vi "Music Visualizer Example.vi"() -> ()   [LabVIEW 2020]
uses:
  <vilib>/Analysis/5stat.llb/RMS (DBL).vi
  <vilib>/sound2/lvsound2.llb/Sound File Info (path).vi
  <vilib>/sound2/lvsound2.llb/Sound File Read Open.vi
  <vilib>/sound2/lvsound2.llb/Sound File Read (DBL).vi
  <vilib>/sound2/lvsound2.llb/Sound Output Write (DBL).vi
  <vilib>/Analysis/NI_AALPro.lvlib
  <vilib>/ptbypt/NI_PtbyPt.lvlib
panel:
  in  "Color Box":u32(colorbox)=5883391
  out "XY Graph":cluster{dbl[], dbl[]}[](graph)
  in  "Stop":bool
  in  "Buffer Size (samples)":i32=2048
  in  "Music File":path
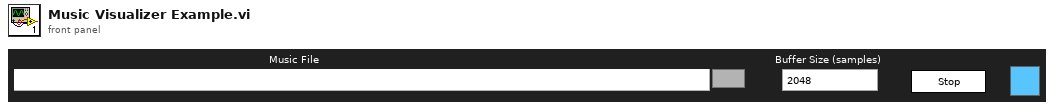
[diagram p1: front panel]
types:
  T1 = typedef "Sound Data Format.ctl" = cluster{"sample rate (S/s)":dbl, "number of channels":i32, "bits per sample":i32}
  T2 = typedef "Sound Output Task ID.ctl" = u32
  T3 = typedef "Sound File Refnum.ctl" = refnum<file>
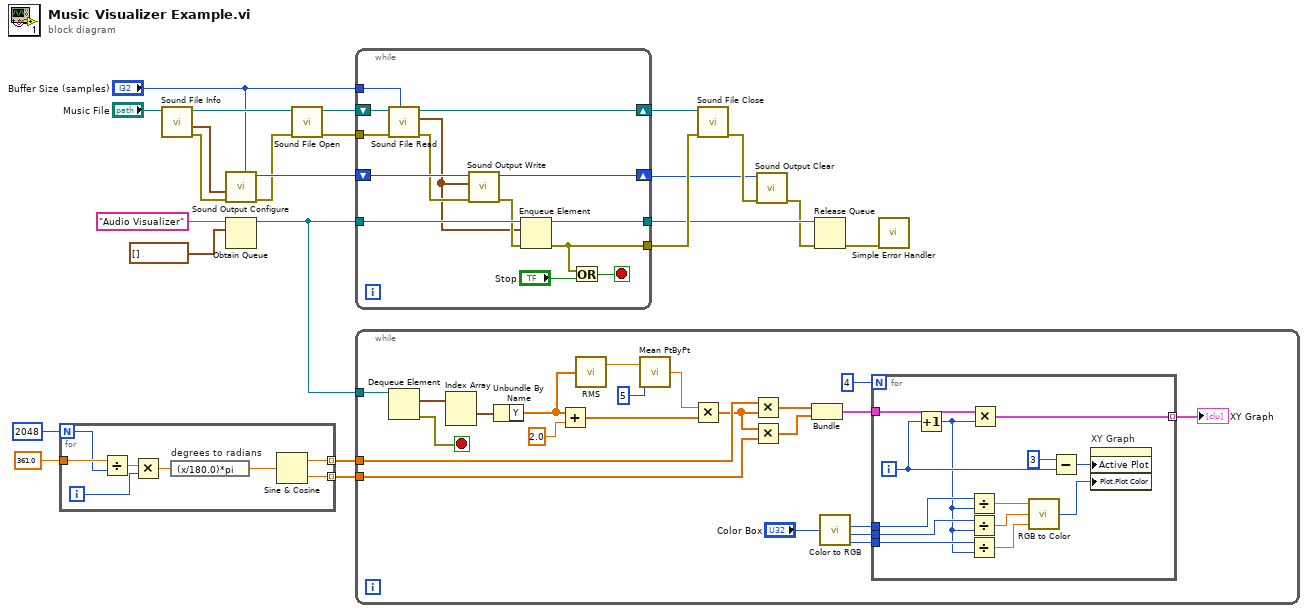
[diagram p0: block diagram]
diagram:
  n1 = for {
    N: 2048 -> [w30]
    tunnel: 361.0 -> [w31]
    tunnel: [w26] -> w2 mode=indexing
    tunnel: [w25] -> w1 mode=indexing
    i -> [w28]
    n2 = Divide(x=w31, y=w30) -> (x/y=w29:dbl)
    n3 = Multiply(x=w29, y=w28) -> (x*y=w27:dbl)
    n4 = expression code="(x/180.0)*pi" "degrees to radians"(w27) -> (w24:dbl)
    n5 = Sine & Cosine(0:w24) -> (1:w26:dbl, 2:w25:dbl)
  }
  n6 = call-poly <vilib>:"Sound File Info.vi"("path"="Music File") -> ("error out"=w6:errorcluster, "sound format"=w13:T1, "path out"=w16:path)  [unwired: 7 in, 1 out]
  n7 = call <vilib>:"Sound Output Configure.vi"("number of samples/ch"="Buffer Size (samples)", "error in (no error)"=w6, "sound format"=w13) -> ("error out"=w5:errorcluster, "task ID"=w11:T2)  [unwired: 7 in]
  n8 = Obtain Queue(name (unnamed)="Audio Visualizer", element data type=waveform(dbl)[] [] ("data")) -> (queue out=w10:refnum<queue>)  [unwired: 3 in, 2 out]
  n9 = call-poly <vilib>:"Sound File Open.vi"("error in (no error)"=w5, "path"=w16) -> ("error out"=w21:errorcluster, "sound file refnum"=w23:T3)  [unwired: 8 in]
  n10 = while {
    tunnel: "Buffer Size (samples)" -> [w44]
    shift-right: [w43] -> w22
    shift-left: w23 -> [w45]
    tunnel: w21 -> [w42]
    tunnel: [w38] -> w20
    tunnel: w10 -> [w39]
    tunnel: [w37] -> w19
    shift-right: [w33] -> w7
    shift-left: w11 -> [w36]
    stop <- w41 stop-if-true
    n11 = call-poly <vilib>:"Sound File Read.vi"("number of samples/ch (-1: all)"=w44, "error in (no error)"=w42, "sound file refnum"=w45) -> ("error out"=w35:errorcluster, "data"=w32:waveform(dbl)[], "sound file refnum out"=w43:T3)  [unwired: 4 in, 2 out]
    n12 = call-poly <vilib>:"Sound Output Write.vi"("error in (no error)"=w35, "data"=w32, "task ID"=w36) -> ("error out"=w34:errorcluster, "task ID out"=w33:T2)  [unwired: 7 in]
    n13 = Enqueue Element(queue=w39, element=w32, error in (no error)=w34) -> (queue out=w37:refnum<queue>, error out=w38:errorcluster)  [unwired: 1 in, 1 out]
    n14 = Or(x=w38, y="Stop") -> (x .or. y?=w41:bool)
  }
  n15 = while {
    tunnel: w10 -> [w67]
    tunnel: w2 -> [w64]
    tunnel: w1 -> [w63]
    stop <- w66 stop-if-true
    n16 = Dequeue Element(queue=w67) -> (element=w65:waveform(dbl)[], error out=w66:errorcluster)  [unwired: 2 in, 2 out]
    n17 = Index Array(array=w65) -> (element #1=w62:waveform(dbl))  [unwired: 2 in, 1 out]
    n18 = Unbundle By Name(w62) -> ("Y"=w46:dbl[])
    n19 = Add(x=w46, y=2.0) -> (x+y=w61:dbl[])
    n20 = call-poly <vilib>:"RMS.vi"("X"=w46) -> ("rms value"=w49:dbl)  [unwired: 1 out]
    n21 = call <vilib>:"Mean PtByPt.vi"("x"=w49, "sample length"=5) -> ("mean"=w48:dbl)  [unwired: 2 in, 1 out]
    n22 = Multiply(x=w48, y=w61) -> (x*y=w50:dbl[])
    n23 = Multiply(x=w64, y=w50) -> (x*y=w59:dbl[])
    n24 = Multiply(x=w50, y=w63) -> (x*y=w58:dbl[])
    n25 = Bundle(w59, w58) -> (w57:cluster{dbl[], dbl[]})  [unwired: 1 in]
    n26 = call <vilib>:"Color to RGB.vi"("Color"="Color Box") -> ("R"=w53:u8, "G"=w52:u8, "B"=w51:u8)  [unwired: 1 out]
    n27 = for {
      N: 4 -> [_]
      tunnel: w57 -> [w80]
      tunnel: [w79] -> w55 mode=indexing
      tunnel: w53 -> [w77]
      tunnel: w52 -> [w76]
      tunnel: w51 -> [w75]
      i -> [w78]
      n28 = Increment(x=w78) -> (x+1=w74:i32)
      n29 = Divide(x=w77, y=w74) -> (x/y=w71:dbl)
      n30 = Divide(x=w76, y=w74) -> (x/y=w70:dbl)
      n31 = Divide(x=w75, y=w74) -> (x/y=w73:dbl)
      n32 = Multiply(x=w80, y=w74) -> (x*y=w79:cluster{dbl[], dbl[]})
      n33 = call <vilib>:"RGB to Color.vi"("B"=w73, "G"=w70, "R"=w71) -> ("Color"=w72:u32)
      n34 = Subtract(x=3, y=w78) -> (x-y=w69:i32)
      n35 = property on="XY Graph" class="XYGraph (strict)"("Active Plot"=w69, "Plot.Plot Color"=w72) -> ()  [unwired: 2 in, 2 out]
    }
    "XY Graph" <- w55
  }
  n36 = call <vilib>:"Sound File Close.vi"("error in (no error)"=w20, "sound file refnum"=w22) -> ("error out"=w9:errorcluster)  [unwired: 9 in]
  n37 = call <vilib>:"Sound Output Clear.vi"("error in (no error)"=w9, "task ID"=w7) -> ("error out"=w8:errorcluster)  [unwired: 9 in]
  n38 = Release Queue(queue=w19, error in (no error)=w8) -> (error out=w18:errorcluster)  [unwired: 1 in, 2 out]
  n39 = call <vilib>:"Simple Error Handler.vi"("error in (no error)"=w18) -> ()  [unwired: 4 in, 5 out]
